vi "ReaderToVariant.vi"(7 "CloseReader":bool=TRUE, 10 "Error In":errorcluster, 11 "Reader":refnum<k24>) -> (2 "Error Out":errorcluster, 3 "Variant":variant, 5 "Read":bool)   [LabVIEW 2020, in "ORM_ADONet.lvlib" / "ADORow.lvclass"]
uses:
  ADORow/ADORow.lvclass
  System.Data
  ADORow/ADORow.lvclass/ADORow.ctl
  <vilib>/Utility/Data Type/NI_Data Type.lvlib
panel:
  out "error out":errorcluster
  out "Array 3":string[](array[string])
  out "Array 2":variant[](array[variant])
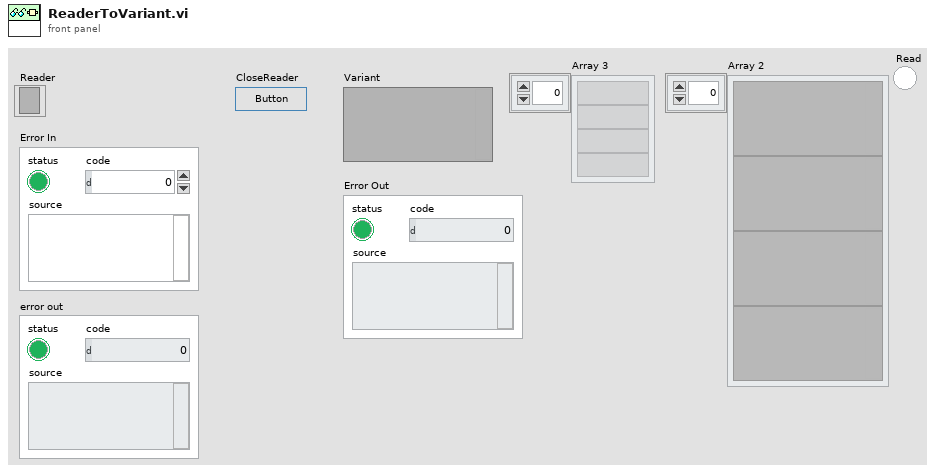
[diagram p1: front panel]
types:
  T1 = typedef "NI_Data Type.lvlib/Data Type.ctl" = enum8{"Invalid Type", "Void", "I8", "I16", "I32", "I64", "U8", "U16", "U32", "U64", "Single Float", "Double Float", "Extended Float", "Single Complex", "Double Complex", "Extended Complex", "Enum U8", "Enum U16", "Enum U32", "Enum U64", "Single Float With Unit", "Double Float With Unit", "Extended Float With Unit", "Single Complex with Unit", "Double Complex with Unit", "Extended Complex with Unit", "Boolean", "String", "Path", "Picture", "Tag", "Array", "Cluster", "Variant", "LV Variant", "Waveform", "Timestamp", "Digital Waveform", "Digital Data", "ExpressData", "Refnum", "External Data", "VI", "Poly VI", "LabVIEW Class Instance", "Fixed Point", "Set Collection", "Map Collection"}
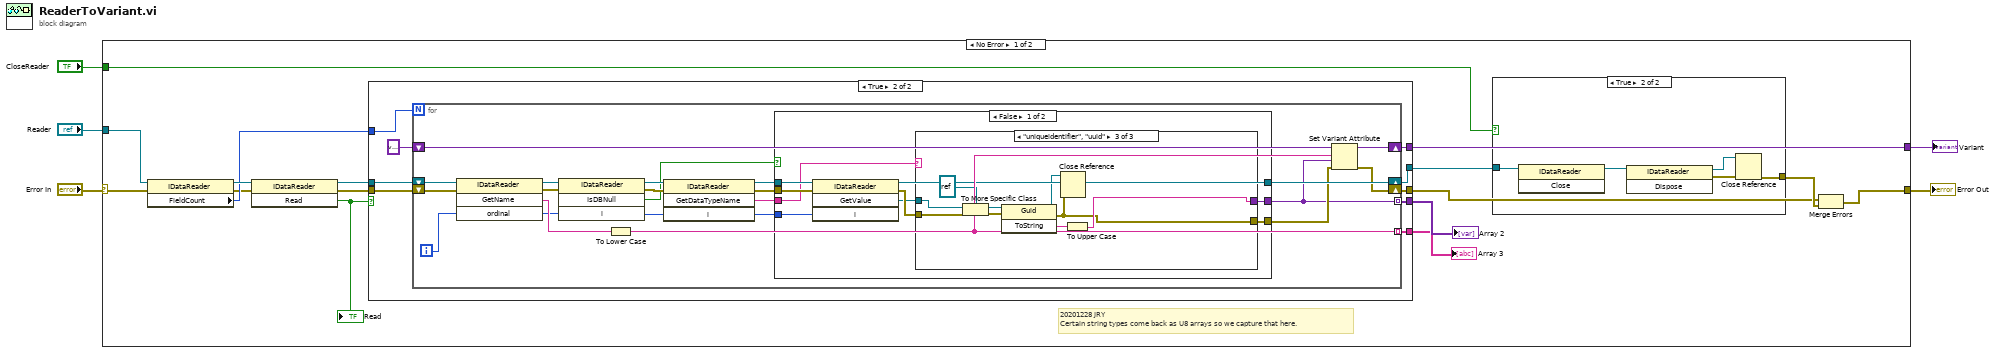
[diagram p0: block diagram]
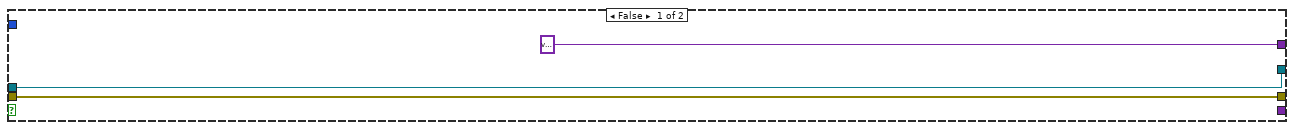
[diagram p2: hidden frame]
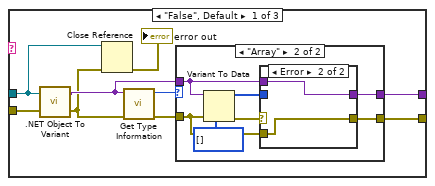
[diagram p3: hidden frame]
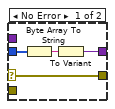
[diagram p5: hidden frame]
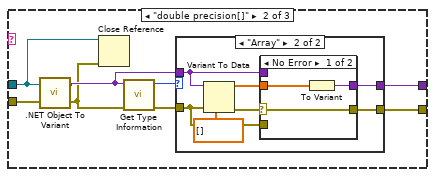
[diagram p6: hidden frame]
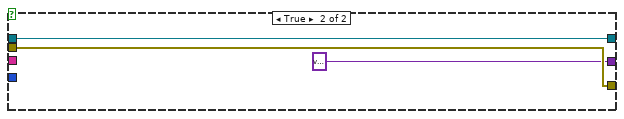
[diagram p9: hidden frame]
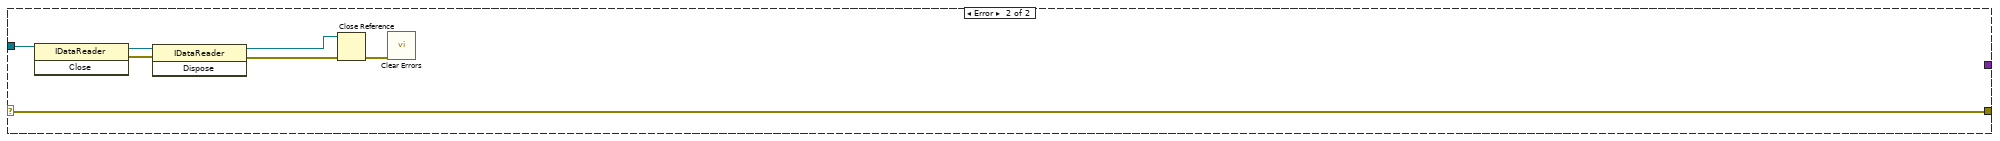
[diagram p11: hidden frame]
diagram:
  n1 = case shown="No Error" "Error In" {
    selector: "Error In" -> [w15 w125]
    tunnel: "Reader" -> [w14 w127]
    tunnel: [w11 _] -> w3
    tunnel: [w9 w125] -> w2
    tunnel: "CloseReader" -> [w6 _]
    frame No Error {
      # "20201228 JRY\nCertain string types come back as U8 arrays so we capture that here."
      n2 = property class="IDataReader"(reference=w14, error in=w15) -> (reference out=w21:refnum<k24>, error out=w13:errorcluster, "FieldCount"=w17:i32)
      n3 = invoke class="IDataReader" method="Read"(reference=w21, error in=w13) -> (reference out=w20:refnum<k24>, error out=w12:errorcluster, "Read"=w7:bool)  [unwired: 1 in]
      "Read" <- w7
      n4 = case shown="True" w7 {
        tunnel: w20 -> [w23 w33]
        tunnel: [w23 w32] -> w19
        tunnel: [_ w31] -> w18
        tunnel: w17 -> [_ w30]
        tunnel: [_ w29] -> w16
        tunnel: w12 -> [w22 w28]
        tunnel: [variant w26] -> w11
        tunnel: [w22 w25] -> w8
        frame False {
        }
        frame True {
          n5 = for {
            N: w30 -> [_]
            shift-right: [w52] -> w32
            shift-left: w33 -> [w51]
            tunnel: [w43] -> w31 mode=indexing
            tunnel: [w42] -> w29 mode=indexing
            shift-right: [w46] -> w25
            shift-left: w28 -> [w50]
            shift-right: [w48] -> w26
            shift-left: variant -> [w49]
            i -> [w35]
            n6 = invoke class="IDataReader" method="GetName"(reference=w51, error in=w50, "ordinal"=w35) -> (reference out=w37:refnum<k24>, error out=w45:errorcluster, "GetName"=w47:string)  [unwired: 1 in, 1 out]
            n7 = invoke class="IDataReader" method="IsDBNull"(reference=w37, error in=w45, "i"=w35) -> (reference out=w36:refnum<k24>, error out=w38:errorcluster, "IsDBNull"=w34:bool)  [unwired: 1 in, 1 out]
            n8 = To Lower Case(string=w47) -> (all lower case string=w42:string)
            n9 = invoke class="IDataReader" method="GetDataTypeName"(reference=w36, error in=w38, "i"=w35) -> (reference out=w40:refnum<k24>, error out=w41:errorcluster, "GetDataTypeName"=w39:string)  [unwired: 1 in, 1 out]
            n10 = case shown="False" w34 {
              tunnel: [w61 w119] -> w52
              tunnel: [w59 w118] -> w44
              tunnel: [w58 variant ("variant")] -> w43
              tunnel: w41 -> [w57 w118]
              tunnel: w40 -> [w56 w119]
              tunnel: w39 -> [w55 _]
              tunnel: w35 -> [w53 _]
              frame False {
                n11 = invoke class="IDataReader" method="GetValue"(reference=w56, error in=w57, "i"=w53) -> (reference out=w61:refnum<k24>, error out=w60:errorcluster, "GetValue"=w54:refnum<k24>)  [unwired: 1 in, 1 out]
                n12 = case shown="\"uniqueidentifier\", \"uuid\"" w55 {
                  tunnel: w54 -> [w63 w87 w115]
                  tunnel: w60 -> [w70 w93 w116]
                  tunnel: [w66 w89 w109] -> w59
                  tunnel: [w65 w88 w110] -> w58
                  frame "False", Default {
                    n13 = call <vilib>:".NET Object To Variant.vi"("error in (no error)"=w70, ".NET object"=w63) -> ("error out"=w64:errorcluster, "variant"=w67:variant)
                    n14 = Close Reference(reference=w63, error in (no error)=w64) -> (error out=→"error out":errorcluster)
                    n15 = call <vilib>:"Get Type Information.vi"("error in (no error)"=w64, "variant"=w67) -> ("error out"=w68:errorcluster, "type"=w69:T1)  [unwired: 5 in, 3 out]
                    n16 = case shown="\"Array\"" w69 {
                      tunnel: w67 -> [w72 w75]
                      tunnel: w68 -> [w71 w74]
                      tunnel: [w72 w77] -> w65
                      tunnel: [w71 w73] -> w66
                      frame "Invalid Type", Default {
                      }
                      frame "Array" {
                        n17 = Variant To Data(error in=w74, type=u8[] [], Variant=w75) -> (data=w78:u8[], error out=w76:errorcluster)
                        n18 = case shown="Error" w76 {
                          selector: w76 -> [w80 _]
                          tunnel: w78 -> [w83 _]
                          tunnel: [w81 w85] -> w77
                          tunnel: w75 -> [_ w85]
                          tunnel: w74 -> [_ w84]
                          tunnel: [w80 w84] -> w73
                          frame No Error {
                            n19 = Byte Array To String(unsigned byte array=w83) -> (string=w82:string)
                            n20 = To Variant(anything=w82) -> (Variant=w81:variant)
                          }
                          frame Error {
                          }
                        }
                      }
                    }
                  }
                  frame "double precision[]" {
                    n21 = call <vilib>:".NET Object To Variant.vi"("error in (no error)"=w93, ".NET object"=w87) -> ("error out"=w86:errorcluster, "variant"=w90:variant)
                    n22 = Close Reference(reference=w87, error in (no error)=w86) -> ()  [unwired: 1 out]
                    n23 = call <vilib>:"Get Type Information.vi"("error in (no error)"=w86, "variant"=w90) -> ("error out"=w91:errorcluster, "type"=w92:T1)  [unwired: 5 in, 3 out]
                    n24 = case shown="\"Array\"" w92 {
                      tunnel: w90 -> [w95 w98]
                      tunnel: w91 -> [w94 w97]
                      tunnel: [w95 w100] -> w88
                      tunnel: [w94 w96] -> w89
                      frame "Invalid Type", Default {
                      }
                      frame "Array" {
                        n25 = Variant To Data(error in=w97, type=dbl[] [], Variant=w98) -> (data=w101:dbl[], error out=w99:errorcluster)
                        n26 = case shown="No Error" w99 {
                          selector: w99 -> [w104 _]
                          tunnel: w101 -> [w103 _]
                          tunnel: [w105 w107] -> w100
                          tunnel: w98 -> [_ w107]
                          tunnel: w97 -> [_ w106]
                          tunnel: [w104 w106] -> w96
                          frame No Error {
                            n27 = To Variant(anything=w103) -> (Variant=w105:variant)
                          }
                          frame Error {
                          }
                        }
                      }
                    }
                  }
                  frame "uniqueidentifier", "uuid" {
                    n28 = To More Specific Class(target class=refnum<k24> refnum ("NewGuid"), reference=w115, error in=w116) -> (specific class reference=w112:refnum<k24>, error out=w113:errorcluster)
                    n29 = invoke class="Guid" method="ToString"(reference=w112, error in=w113) -> (reference out=w108:refnum<k24>, error out=w109:errorcluster, "ToString"=w111:string)  [unwired: 1 in]
                    n30 = Close Reference(reference=w108, error in (no error)=w109) -> ()  [unwired: 1 out]
                    n31 = To Upper Case(1:w111) -> (0:w110:string)
                  }
                }
              }
              frame True {
              }
            }
            n32 = Set Variant Attribute(Variant=w49, name=w42, value=w43, error in=w44) -> (Variant out=w48:variant, error out=w46:errorcluster)  [unwired: 1 out]
          }
        }
      }
      "Array 2" <- w18
      "Array 3" <- w16
      n33 = case shown="True" w6 {
        tunnel: w19 -> [_ w121]
        tunnel: [_ w120] -> w10
        frame False {
        }
        frame True {
          n34 = invoke class="IDataReader" method="Close"(reference=w121) -> (reference out=w124:refnum<k24>)  [unwired: 2 in, 2 out]
          n35 = invoke class="IDataReader" method="Dispose"(reference=w124) -> (reference out=w122:refnum<k24>, error out=w123:errorcluster)  [unwired: 2 in, 1 out]
          n36 = Close Reference(reference=w122, error in (no error)=w123) -> (error out=w120:errorcluster)
        }
      }
      n37 = Merge Errors(w8, w10) -> (w9:errorcluster)
    }
    frame Error {
      n38 = invoke class="IDataReader" method="Close"(reference=w127) -> (reference out=w131:refnum<k24>, error out=w130:errorcluster)  [unwired: 2 in, 1 out]
      n39 = invoke class="IDataReader" method="Dispose"(reference=w131, error in=w130) -> (reference out=w128:refnum<k24>, error out=w129:errorcluster)  [unwired: 1 in, 1 out]
      n40 = Close Reference(reference=w128, error in (no error)=w129) -> (error out=w126:errorcluster)
      n41 = call <vilib>:"Clear Errors.vi"("error in (no error)"=w126) -> ()  [unwired: 5 in, 2 out]
    }
  }
  "Error Out" <- w2
  "Variant" <- w3
